vi "Write Local Msg Set.vi"(11 "Base Actor in":refnum<class "Base Actor.lvclass">) -> (3 "Base Actor out":refnum<class "Base Actor.lvclass">)   [LabVIEW 2025, in "jettl.lvlib" / "Actor.lvlib" / "Base Actor.lvclass"]
uses:
  Base Actor.lvclass
  Base Actor.lvclass/Base Actor.ctl
  Actor.lvlib
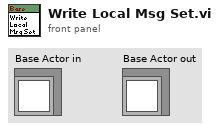
[diagram p1: front panel]
types:
  T1 = typedef "jettl.lvlib/Actor.lvlib/Msg Set.ctl" = set{refnum<class "Msg.lvclass">}
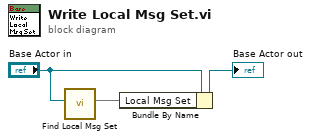
[diagram p0: block diagram]
diagram:
  n1 = call "Find Local Msg Set.vi"("Variant (X Actor.lvclass)"="Base Actor in") -> ("Local Msg Set"=w2:T1)  [unwired: 10 in]
  n2 = Bundle By Name(cluster="Base Actor in", "Local Msg Set"=w2) -> (→"Base Actor out":refnum<class "Base Actor.lvclass">)
